vi "SAOMM-LUT2XML.vi"(0 "XMLPath":path, 7 "CompleteLUT":dbl[][](array[numeric])) -> ()   [LabVIEW 2011]
uses:
  <vilib>/xml/Close Reference(Node).vi
  <vilib>/xml/NI_XML.lvlib
  Program Files (x86)/National Instruments/LabVIEW 2011/resource/objmgr/DOMUserDefRef.rc
panel:
  out "Array":dbl[](array[numeric])
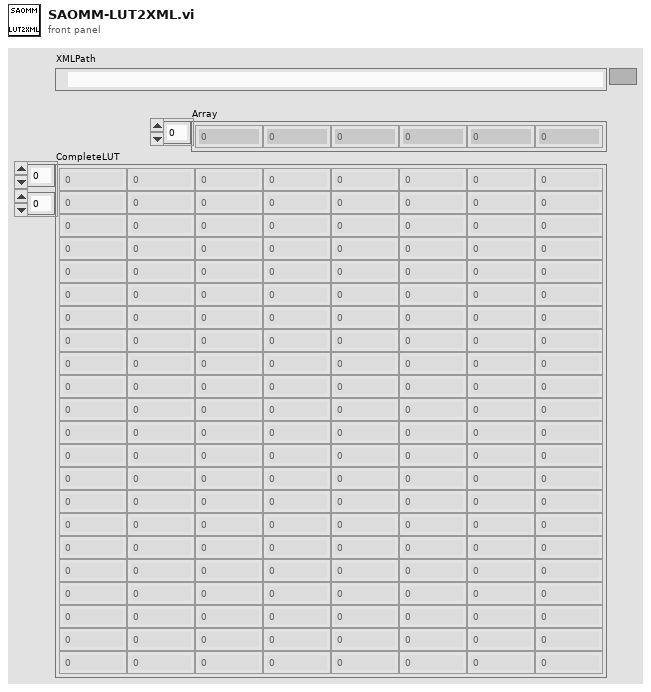
[diagram p1: front panel]
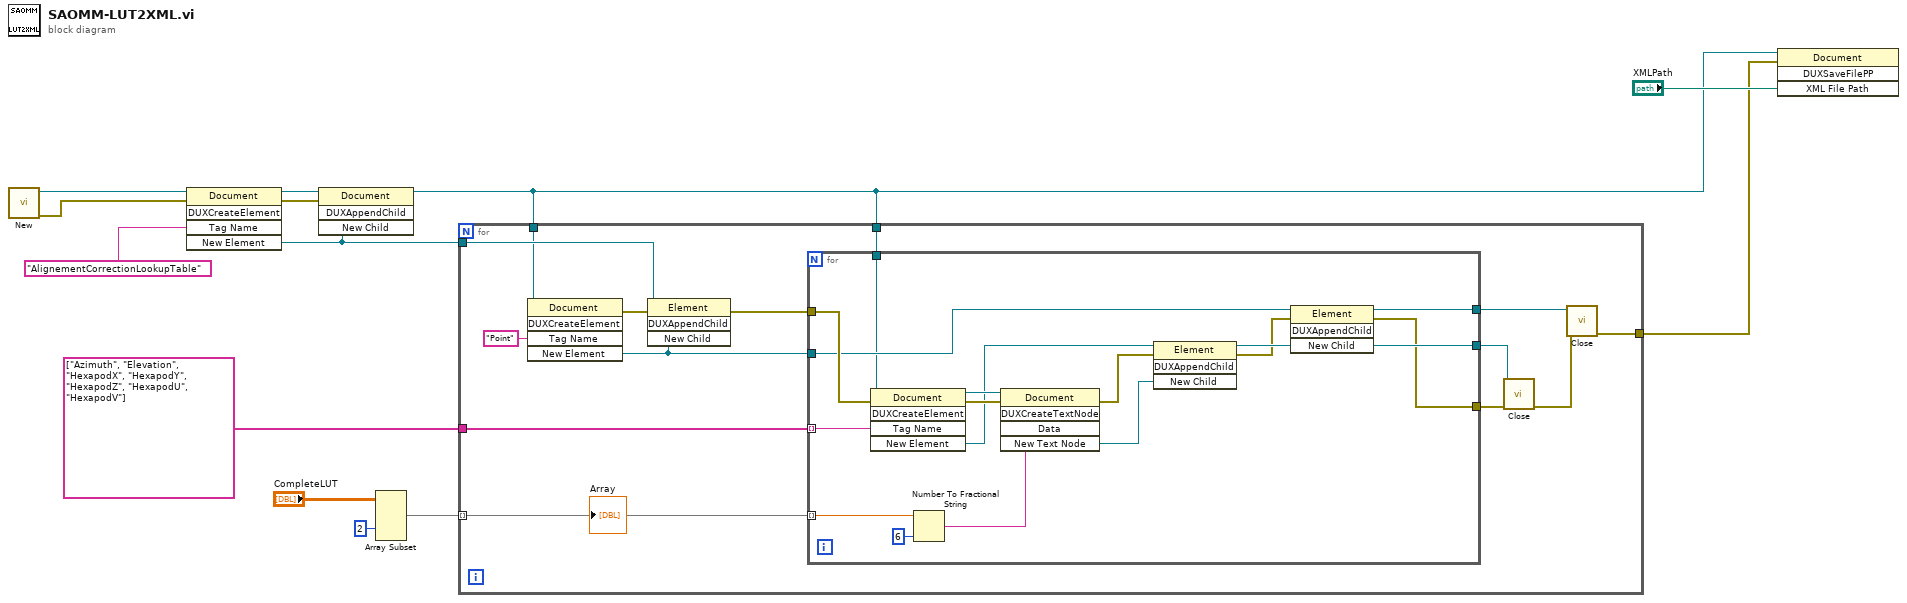
[diagram p0: block diagram]
diagram:
  n1 = call <vilib>:"New.vi"() -> ("error out"=w9:errorcluster, "DOM document out"=w13:refnum<k20>)  [unwired: 8 in]
  n2 = invoke class="Document" method="DUXCreateElement"(reference=w13, error in=w9, "Tag Name"="AlignementCorrectionLookupTable") -> (reference out=w11:refnum<k20>, error out=w8:errorcluster, "New Element"=w4:refnum<k20>)  [unwired: 2 in, 2 out]
  n3 = invoke class="Document" method="DUXAppendChild"(reference=w11, error in=w8, "New Child"=w4) -> (reference out=w1:refnum<k20>)  [unwired: 1 in, 3 out]
  n4 = Array Subset(array="CompleteLUT", index (col)=2 ("index")) -> (w6:dbl[][])  [unwired: 3 in]
  n5 = for {
    tunnel: string[] ["Azimuth", "Elevation", "HexapodX", "HexapodY", "HexapodZ", "HexapodU", "HexapodV"] -> [w24]
    tunnel: w6 -> [w23] mode=indexing
    tunnel: w4 -> [w22]
    tunnel: w1 -> [w20]
    tunnel: w1 -> [w19]
    tunnel: [w14] -> w2
    n6 = invoke class="Document" method="DUXCreateElement"(reference=w20, "Tag Name"="Point") -> (error out=w26:errorcluster, "New Element"=w21:refnum<k20>)  [unwired: 3 in, 3 out]
    n7 = invoke class="Element" method="DUXAppendChild"(reference=w22, error in=w26, "New Child"=w21) -> (error out=w25:errorcluster)  [unwired: 1 in, 3 out]
    n8 = for {
      tunnel: w25 -> [w41]
      tunnel: w24 -> [w40] mode=indexing
      tunnel: w23 -> [w39] mode=indexing
      tunnel: w21 -> [w35]
      tunnel: w19 -> [w34]
      tunnel: [w32] -> w18
      tunnel: [w31] -> w17
      tunnel: [w28] -> w16
      n9 = invoke class="Document" method="DUXCreateElement"(reference=w34, error in=w41, "Tag Name"=w40) -> (reference out=w42:refnum<k20>, error out=w43:errorcluster, "New Element"=w33:refnum<k20>)  [unwired: 2 in, 2 out]
      n10 = Number To Fractional String(number=w39, precision (6)=i16 6) -> (F-format string=w37:string)  [unwired: 2 in]
      n11 = invoke class="Document" method="DUXCreateTextNode"(reference=w42, error in=w43, "Data"=w37) -> (error out=w30:errorcluster, "New Text Node"=w36:refnum<k20>)  [unwired: 2 in, 3 out]
      n12 = invoke class="Element" method="DUXAppendChild"(reference=w33, error in=w30, "New Child"=w36) -> (reference out=w31:refnum<k20>, error out=w29:errorcluster)  [unwired: 1 in, 2 out]
      n13 = invoke class="Element" method="DUXAppendChild"(reference=w35, error in=w29, "New Child"=w31) -> (reference out=w32:refnum<k20>, error out=w28:errorcluster)  [unwired: 1 in, 2 out]
    }
    n14 = call-poly <vilib>:"Close.vi"("error in (no error)"=w16, "node"=w17) -> ("error out"=w15:errorcluster)  [unwired: 7 in]
    n15 = call-poly <vilib>:"Close.vi"("error in (no error)"=w15, "node"=w18) -> ("error out"=w14:errorcluster)  [unwired: 7 in]
    "Array" <- w23
  }
  n16 = invoke class="Document" method="DUXSaveFilePP"(reference=w1, error in=w2, "XML File Path"="XMLPath") -> ()  [unwired: 1 in, 4 out]
